vi "PLS Main.vi"() -> ()   [LabVIEW 2014]
doc: "This Continuous Measurement sample project is based on the Queued Message Handler template.\n\nThe Event Handling Loop generates messages based on user interface actions.\n\nThe Message Handling Loop processes messages generated by the Event Handling Loop, or by other messages. There are also Acquisition and Logging message handling loop subVIs, and a chart updating loop."
uses:
  Digital Control/type de test.ctl
  Settings/Settings.ctl
  Acquisition/Hardware Configuration.ctl
  Settings/conversion.ctl
  Logging/Logging Configuration.ctl
  Generation/Hardware Configuration.ctl
  Digital Control/Hardware Configuration.ctl
  controls/PLS UI Data.ctl
  controls/PLS UI State.ctl
  Acquisition/GLB_compteurs.vi
  support/Message Queue/Enqueue Message (Single).vi
  support/GLB_PAmonts.vi
  Digital Control/GLB_Timing.vi
  Acquisition/GLB_Fsave.vi
  support/Message Queue/Enqueue Message (Array).vi
  <vilib>/Utility/error.llb/Error Cluster From Error Code.vi
  <vilib>/ErrorRing/Error Ring.xnode
  Acquisition/PLS Acquisition.lvlib
  Logging/PLS Logging.lvlib
  Settings/PLS Settings.lvlib
  support/User Event - Stop/PLS User Event - Stop.lvlib
  support/Message Queue/PLS Message Queue.lvlib
  Generation/PLS Generation.lvlib
  Digital Control/PLS Digital Control.lvlib
panel:
  in  "Tab":enum32{"Mode manuel", "Lancement cycle"}(tab)
  out "Data":waveform(dbl)[](graph)
  in  "p0.2":bool caption="Eau froide"
  in  "p0.3":bool caption="Eau chaude"
  in  "p0.5":bool caption="Coup de bélier"
  out "compteurs":T1 {"Ligne 4" format="%#.3f l/min"; "Ligne 3" format="%#.3f l/min"; "Ligne 2" format="%#.3f l/min"; "c0" format="%#.3f l/min"}
  in  "Start":bool
  in  "Stop":bool
  in  "Settings":bool
  in  "L4_Twarm":dbl=5.0 caption="Période chaude" min=5.0 max=1000.0 step=0.1 format="%d s"
  in  "L4_Tcold":dbl=5.0 caption="Période froide" min=5.0 max=1000.0 step=0.1 format="%d s"
  in  "L4_Tcons":dbl=30.0 caption="T consigne" min=10.0 max=80.0 step=1.0 format="%#.1f °C"
  in  "L4_stop":bool
  in  "L4_start":bool
  in  "L4_file":path caption="Fichier de sortie"
  in  "L4_fsave":i32(ring)=10 caption="Fréquence enregistrement" items=["1 kHz"=10, "100 Hz"=100, "10 Hz"=1000, "1 Hz"=10000]
  out "Temp":dbl(slide) caption="Température" scale=0.0..100.0
  out "L4_Vtot":dbl caption="Volume total" format="%#.1f l"
  out "L4_debit":dbl(knob) caption="Débit" scale=0.0..15.0
  out "L4_Pfiltre":dbl(knob) caption="Pression filtre" scale=0.0..10.0
  in  "L4_Pamont":dbl=1.0 caption="Pression amont" min=0.0 max=10.0 step=0.1 format="%#.1f Bar"
  in  "Type de test":T2
  out "L3_Vtot":dbl caption="Volume total" format="%#.1f l"
  in  "L3_stop":bool
  in  "L3_start":bool
  in  "L3_file":path caption="Fichier de sortie"
  in  "L3_fsave":i32(ring)=10 caption="Fréquence enregistrement" items=["1 kHz"=10, "100 Hz"=100, "10 Hz"=1000, "1 Hz"=10000]
  out "L3_debit":dbl(knob) caption="Débit" scale=0.0..15.0
  out "L3_Pfiltre":dbl(knob) caption="Pression filtre" scale=0.0..10.0
  in  "L3_Pamont":dbl=1.0 caption="Pression amont" min=0.0 max=10.0 step=0.1 format="%#.1f Bar"
  out "L2_Vtot":dbl caption="Volume total" format="%#.1f l"
  in  "L2_stop":bool
  in  "L2_start":bool
  in  "L2_file":path caption="Fichier de sortie"
  in  "L2_fsave":i32(ring)=10 caption="Fréquence enregistrement" items=["1 kHz"=10, "100 Hz"=100, "10 Hz"=1000, "1 Hz"=10000]
  out "L2_debit":dbl(knob) caption="Débit" scale=0.0..15.0
  out "L2_Pfiltre":dbl(knob) caption="Pression filtre" scale=0.0..10.0
  in  "L2_Pamont":dbl=1.0 caption="Pression amont" min=0.0 max=10.0 step=0.1 format="%#.1f Bar"
  in  "L1_stop":bool
  in  "L1_start":bool
  in  "L1_file":path caption="Fichier de sortie"
  in  "L1_fsave":i32(ring)=10 caption="Fréquence enregistrement" items=["1 kHz"=10, "100 Hz"=100, "10 Hz"=1000, "1 Hz"=10000]
  in  "L1_Tclose":dbl=5.0 caption="Période fermeture" min=5.0 max=1000.0 step=0.1 format="%d s"
  in  "L1_Topen":dbl=5.0 caption="Période ouverture" min=5.0 max=1000.0 step=0.1 format="%d s"
  out "L1_debit":dbl(knob) caption="Débit" scale=0.0..25.0
  out "L1_Pfiltre":dbl(knob) caption="Pression filtre" scale=0.0..15.0
  in  "L1_Pamont":dbl=1.0 caption="Pression amont" min=0.0 max=10.0 step=0.1 format="%#.1f Bar"
  out "soft":string
  # "Ligne 1"
  # "Ligne 2"
  # "Ligne 3"
  # "Ligne 4"
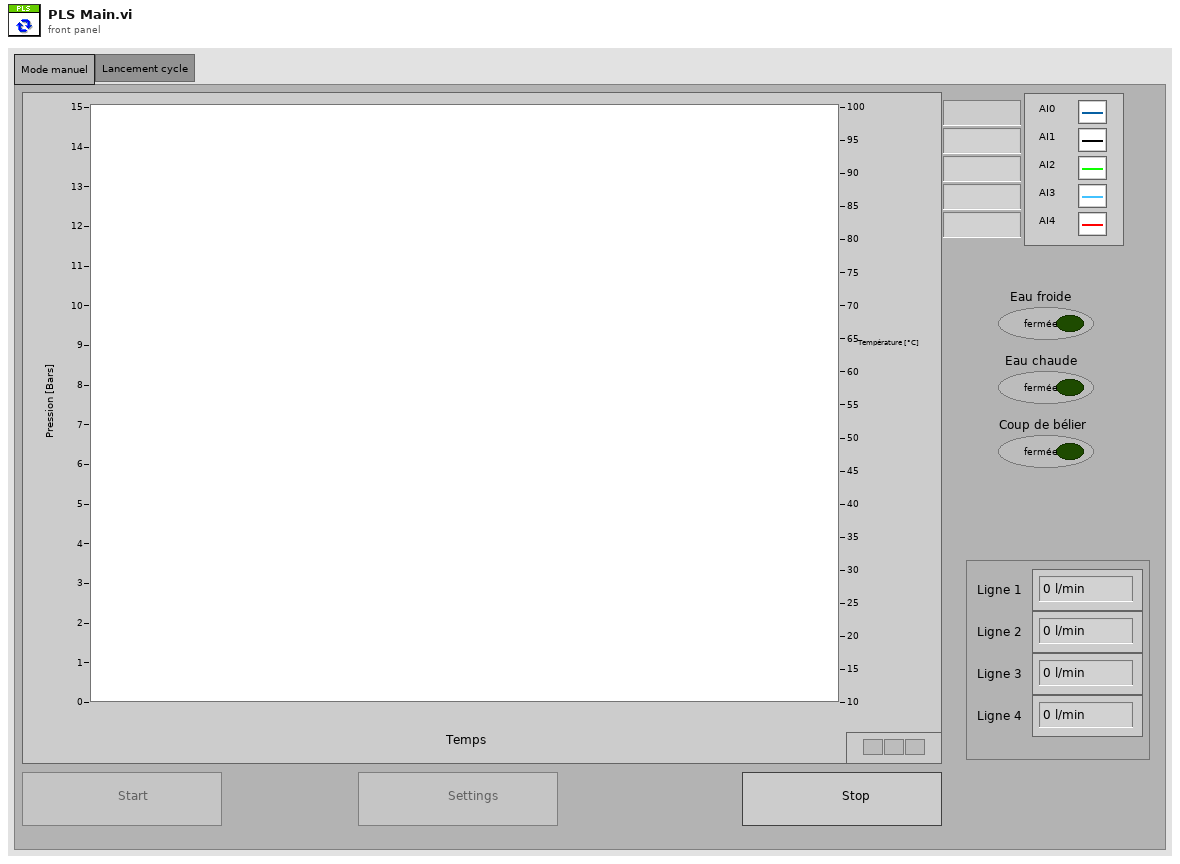
[diagram p1: front panel]
types:
  T1 = cluster{"c0":dbl, "Ligne 2":dbl, "Ligne 3":dbl, "Ligne 4":dbl}
  T2 = typedef "type de test.ctl" = enum16{"Eau froide - standard", "Eau chaude", "Chocs thermiques"}
  T3 = typedef "PLS UI State.ctl" = enum16{"Idle", "Acquiring and Logging", "Waiting for Exit", "Waiting for Exit (Acq Stopped)", "Waiting for Exit (Log Stopped)", "Waiting for Stop", "Waiting for Stop (Acq Stopped)", "Waiting for Stop (Log Stopped)"}
  T4 = typedef "PLS UI Data.ctl" = cluster{"Data Ref":refnum<vi>, "Settings Ref":refnum<vi>, "stop":cluster{"man":refnum<vi>, "L1":refnum<vi>, "L2":refnum<vi>, "L3":refnum<vi>, "L4":refnum<vi>}, "start":cluster{"man":refnum<vi>, "L1":refnum<vi>, "L2":refnum<vi>, "L3":refnum<vi>, "L4":refnum<vi>}, "file":cluster{"L1":refnum<vi>, "L2":refnum<vi>, "L3":refnum<vi>, "L4":refnum<vi>}, "pamont":cluster{"L1":refnum<vi>, "L2":refnum<vi>, "L3":refnum<vi>, "L4":refnum<vi>}, "Fsave":cluster{"L1_fsave":refnum<vi>, "L2_fsave":refnum<vi>, "L3_fsave":refnum<vi>, "L4_fsave":refnum<vi>}, "Tvanne":cluster{"open":refnum<vi>, "close":refnum<vi>}, "Ttemp":cluster{"cold":refnum<vi>, "warm":refnum<vi>}, "temp":refnum<vi>, "Type":refnum<vi>}
  T5 = typedef "PLS Settings.lvlib/Settings.ctl" = cluster{"Acquisition Settings":T6, "Logging Configuration":T8, "Generation Settings":T9, "Digital Control Configuration":T10}
  T6 = typedef "PLS Acquisition.lvlib/Hardware Configuration.ctl" = cluster{"AI":cluster{"task name":string, "task_ref":refnum<k21>, "physical channels":tag, "channels config":cluster{"input terminal configuration":i32, "minimum value":dbl, "maximum value":dbl}, "rate":dbl}, "conversions":cluster{"ai0":T7, "ai1":T7, "ai2":T7, "ai3":T7, "ai4":T7}, "compteur 0":cluster{"task name":string, "task_ref":refnum<k21>, "ctr":tag, "coeff":dbl}, "compteur 1":cluster{"task name":string, "task_ref":refnum<k21>, "ctr":tag, "coeff":dbl}, "compteur 2":cluster{"task name":string, "task_ref":refnum<k21>, "ctr":tag, "coeff":dbl}, "compteur 3":cluster{"task name":string, "task_ref":refnum<k21>, "ctr":tag, "coeff":dbl}}
  T7 = typedef "PLS Settings.lvlib/conversion.ctl" = cluster{"a":dbl, "b":dbl}
  T8 = typedef "PLS Logging.lvlib/Logging Configuration.ctl" = cluster{"Log File Base Path":path, "L1":cluster{"ref":refnum<file>, "actif?":bool, "Fsave":i32}, "L2":cluster{"ref":refnum<file>, "actif?":bool, "Fsave":i32}, "L3":cluster{"ref":refnum<file>, "actif?":bool, "Fsave":i32}, "L4":cluster{"ref":refnum<file>, "actif?":bool, "Fsave":i32}}
  T9 = typedef "PLS Generation.lvlib/Hardware Configuration.ctl" = cluster{"AO":cluster{"task name":string, "task_ref":refnum<k21>, "physical channels":tag}, "PID":cluster{"P":dbl, "I":dbl, "D":dbl}, "conversions":cluster{"ao0":T7}, "setpoint":dbl}
  T10 = typedef "PLS Digital Control.lvlib/Hardware Configuration.ctl" = cluster{"DO":cluster{"task name":string, "task_ref":refnum<k21>, "lines":tag}}
  T11 = typedef "PLS Message Queue.lvlib/All Message Queues.ctl" = cluster{"UI":refnum<queue>, "Acquisition":refnum<queue>, "Logging":refnum<queue>, "Generation":refnum<queue>, "Digital":refnum<queue>}
  T12 = enum8{"Enabled", "Disabled", "Disabled and Grayed Out"}
  T13 = cluster{"L1_Pamont":dbl, "L2_Pamont":dbl, "L3_Pamont":dbl, "L4_Pamont":dbl}
  T14 = cluster{"L1_fsave":i32, "L2_fsave":i32, "L3_fsave":i32, "L4_fsave":i32}
  T15 = enum16{"Eau froide - standard", "Eau chaude", "Chocs thermiques"}
  T16 = cluster{"Stop":refnum<vi>, "L1_stop":refnum<vi>, "L2_stop":refnum<vi>, "L3_stop":refnum<vi>, "L4_stop":refnum<vi>}
  T17 = cluster{"Start":refnum<vi>, "L1_start":refnum<vi>, "L2_start":refnum<vi>, "L3_start":refnum<vi>, "L4_start":refnum<vi>}
  T18 = cluster{"L1_Pamont":refnum<vi>, "L2_Pamont":refnum<vi>, "L3_Pamont":refnum<vi>, "L4_Pamont":refnum<vi>}
  T19 = cluster{"L1_file":refnum<vi>, "L2_file":refnum<vi>, "L3_file":refnum<vi>, "L4_file":refnum<vi>}
  T20 = cluster{"L1_fsave":refnum<vi>, "L2_fsave":refnum<vi>, "L3_fsave":refnum<vi>, "L4_fsave":refnum<vi>}
  T21 = cluster{"L1_Topen":refnum<vi>, "L1_Tclose":refnum<vi>}
  T22 = cluster{"L4_Tcold":refnum<vi>, "L4_Twarm":refnum<vi>}
  T23 = cluster{"man":refnum<vi>, "L1":refnum<vi>, "L2":refnum<vi>, "L3":refnum<vi>, "L4":refnum<vi>}
  T24 = typedef "PLS Logging.lvlib/start info.ctl" = cluster{"path":path, "Fsave":i32, "#ligne":i32}
  T25 = typedef "start info.ctl" = cluster{"type":T2, "ligne index":i32}
  T26 = cluster{"L1":refnum<vi>, "L2":refnum<vi>, "L3":refnum<vi>, "L4":refnum<vi>}
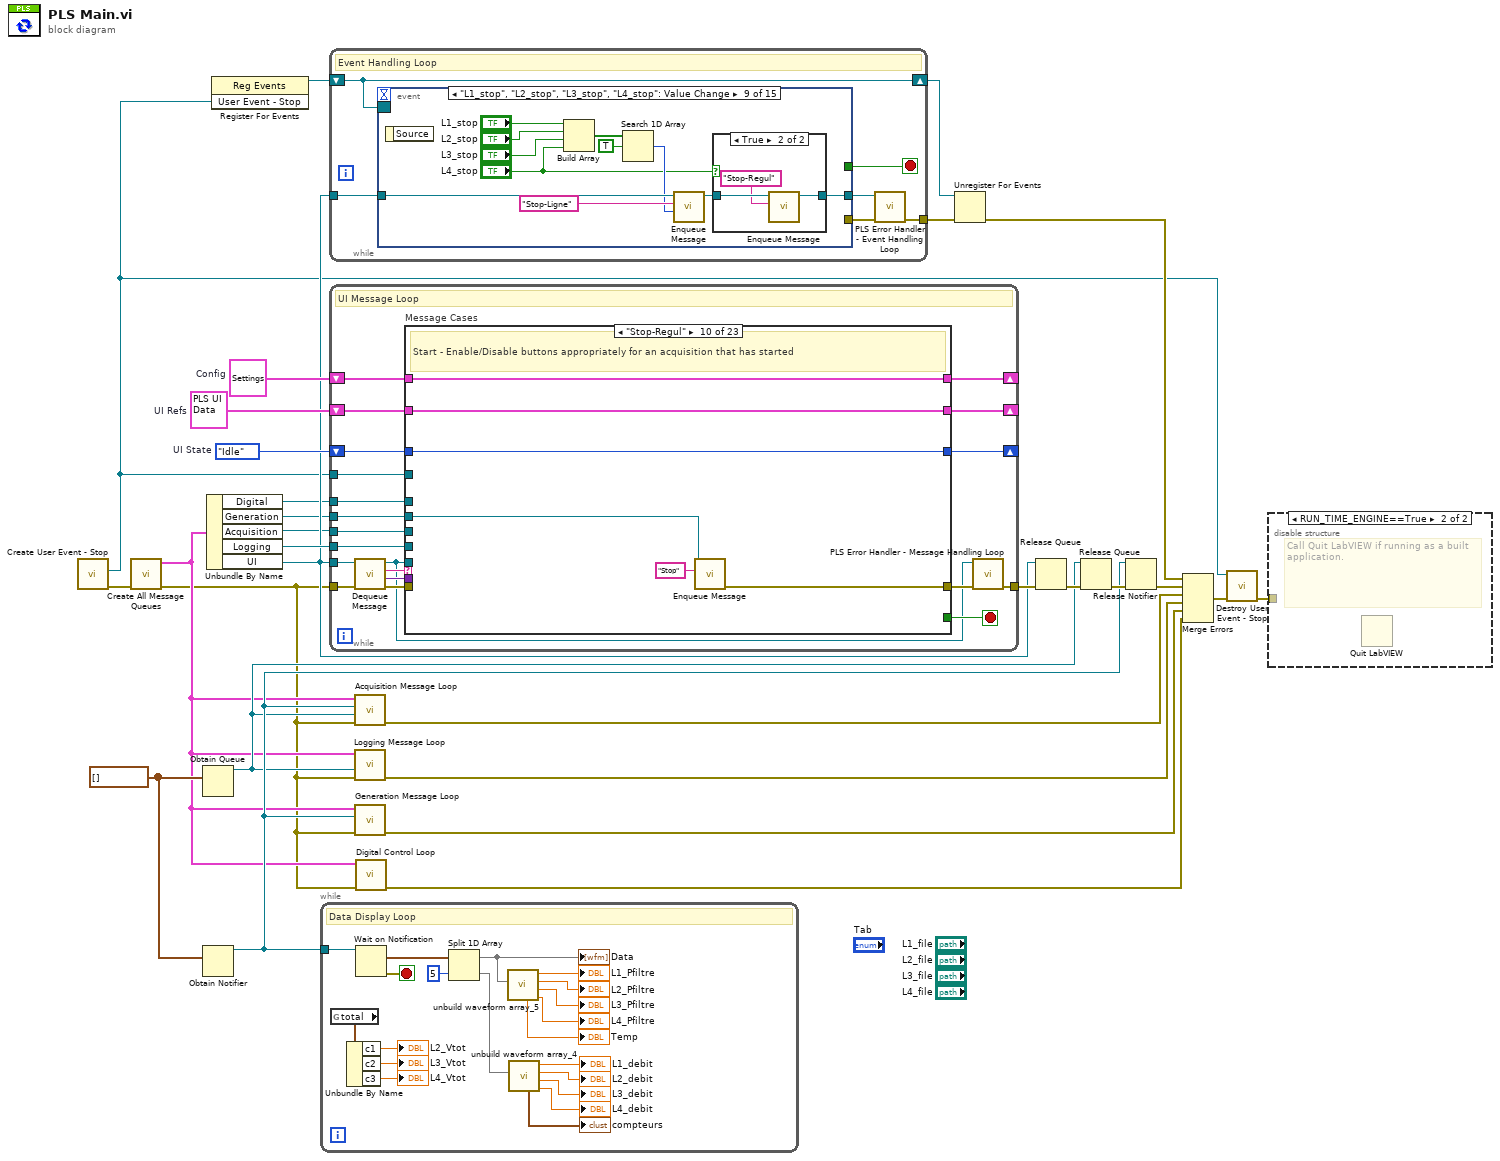
[diagram p0: block diagram]
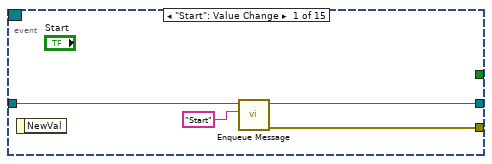
[diagram p3: hidden frame]
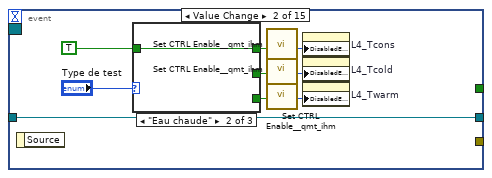
[diagram p4: hidden frame]
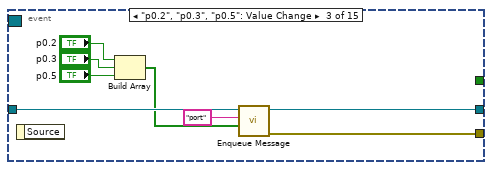
[diagram p7: hidden frame]
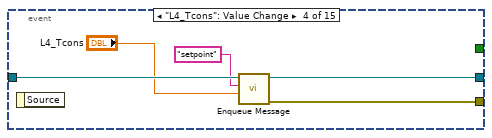
[diagram p8: hidden frame]
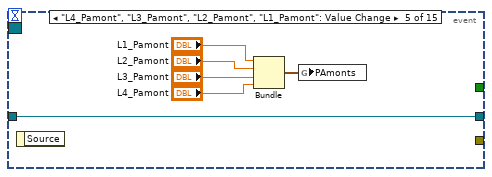
[diagram p9: hidden frame]
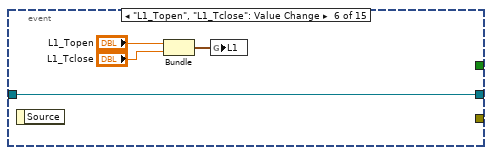
[diagram p10: hidden frame]
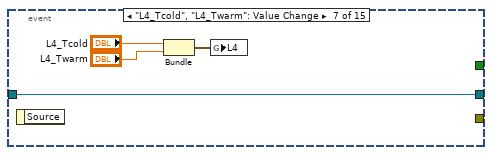
[diagram p11: hidden frame]
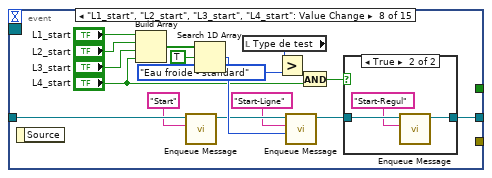
[diagram p12: hidden frame]
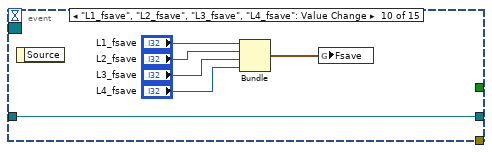
[diagram p15: hidden frame]
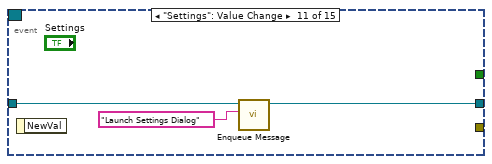
[diagram p16: hidden frame]
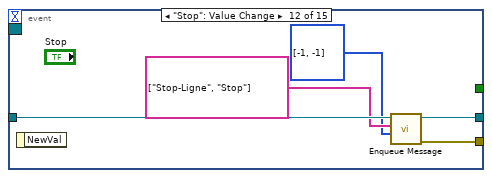
[diagram p17: hidden frame]
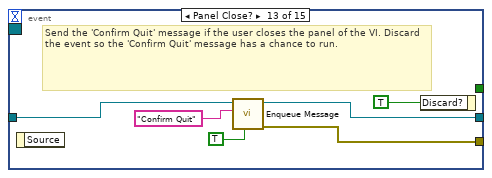
[diagram p18: hidden frame]
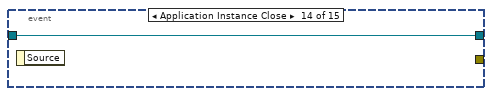
[diagram p19: hidden frame]
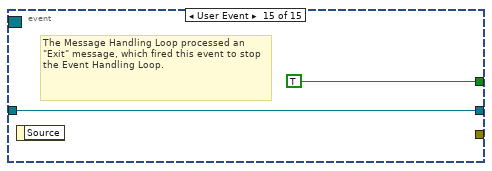
[diagram p20: hidden frame]
diagram:
  w20 = PLS_UI_State."Idle"  # UI State
  w13 = waveform(dbl)[] []
  w22 = T4 {"Data Ref"=refnum, "Settings Ref"=refnum, "stop"={"man"=refnum, "L1"=refnum, "L2"=refnum, "L3"=refnum, "L4"=refnum}, "start"={"man"=refnum, "L1"=refnum, "L2"=refnum, "L3"=refnum, "L4"=refnum}, "file"={"L1"=refnum, "L2"=refnum, "L3"=refnum, "L4"=refnum}, "pamont"={"L1"=refnum, "L2"=refnum, "L3"=refnum, "L4"=refnum}, "Fsave"={"L1_fsave"=refnum, "L2_fsave"=refnum, "L3_fsave"=refnum, "L4_fsave"=refnum}, "Tvanne"={"open"=refnum, "close"=refnum}, "Ttemp"={"cold"=refnum, "warm"=refnum}, "temp"=refnum, "Type"=refnum}  # UI Refs
  w25 = T5 {"Acquisition Settings"={"AI"={"task name"="AI", "task_ref"="", "physical channels"="Dev1/ai0:7", "channels config"={"input terminal configuration"=10106, "minimum value"=-5.0, "maximum value"=5.0}, "rate"=1000.0}, "conversions"={"ai0"={"a"=0.0, "b"=0.0}, "ai1"={"a"=0.0, "b"=0.0}, "ai2"={"a"=0.0, "b"=0.0}, "ai3"={"a"=0.0, "b"=0.0}, "ai4"={"a"=0.0, "b"=0.0}}, "compteur 0"={"task name"="CTR", "task_ref"="", "ctr"="Dev1/ctr0:3", "coeff"=4000.0}, "compteur 1"={"task name"="CTR1", "task_ref"="", "ctr"="Dev1/ctr1", "coeff"=4000.0}, "compteur 2"={"task name"="CTR2", "task_ref"="", "ctr"="Dev1/ctr2", "coeff"=4000.0}, "compteur 3"={"task name"="CTR3", "task_ref"="", "ctr"="Dev1/ctr3", "coeff"=4000.0}}, "Logging Configuration"={"Log File Base Path"=path "", "L1"={"ref"=refnum, "actif?"=FALSE, "Fsave"=0}, "L2"={"ref"=refnum, "actif?"=FALSE, "Fsave"=0}, "L3"={"ref"=refnum, "actif?"=FALSE, "Fsave"=0}, "L4"={"ref"=refnum, "actif?"=FALSE, "Fsave"=0}}, "Generation Settings"={"AO"={"task name"="AO", "task_ref"="", "physical channels"="Dev1/ao0"}, "PID"={"P"=0.0, "I"=0.0, "D"=0.0}, "conversions"={"ao0"={"a"=0.0, "b"=0.0}}, "setpoint"=0.0}, "Digital Control Configuration"={"DO"={"task name"="DO", "task_ref"="", "lines"="Dev1/port0/line2:3, Dev1/port0/line5"}}}  # Config
  n1 = call "Create User Event - Stop.vi"() -> ("error out"=w26:errorcluster, "User Event - Stop"=w1:refnum<user-event>)  [unwired: 10 in]
  n2 = call "Create All Message Queues.vi"("error in (no error)"=w26) -> ("error out"=w3:errorcluster, "Message Queues out"=w4:T11)  [unwired: 9 in]
  n3 = Obtain Queue(element data type=w13) -> (queue out=w11:refnum<queue>)  [unwired: 4 in, 2 out]
  n4 = Obtain Notifier(notification data type=w13) -> (notifier out=w12:refnum<notifier>)  [unwired: 3 in, 2 out]
  n5 = Unbundle By Name(w4) -> ("Digital"=w5:refnum<queue>, "Generation"=w6:refnum<queue>, "Acquisition"=w7:refnum<queue>, "Logging"=w21:refnum<queue>, "UI"=w18:refnum<queue>)
  n6 = register-events(w1) -> (reference out=w10:refnum<event-registration>)  [unwired: 2 in, 1 out]
  n7 = while "Data Display Loop" {
    tunnel: w12 -> [w49]
    stop <- w48 stop-if-true
    # "Data Display Loop"
    n8 = global read "GLB_compteurs.vi" "total"() -> (w33:cluster{"c0":dbl, "c1":dbl, "c2":dbl, "c3":dbl})
    n9 = Unbundle By Name(w33) -> ("c1"=→"L2_Vtot":dbl, "c2"=→"L3_Vtot":dbl, "c3"=→"L4_Vtot":dbl)
    n10 = Wait on Notification(notifier=w49) -> (notification=w46:waveform(dbl)[], error out=w48:errorcluster)  [unwired: 3 in, 2 out]
    n11 = Split 1D Array(array=w46, index=5) -> (first subarray=w42:waveform(dbl)[], second subarray=w39:waveform(dbl)[])
    "Data" <- w42
    n12 = call "unbuild waveform array_5.vi"("Array"=w42) -> ("l4"=→"L4_Pfiltre":dbl, "l3"=→"L3_Pfiltre":dbl, "l2"=→"L2_Pfiltre":dbl, "l1"=→"L1_Pfiltre":dbl, "t"=→"Temp":dbl)  [unwired: 6 in]
    n13 = call "unbuild waveform array_4.vi"("Array"=w39) -> ("4"=→"L4_debit":dbl, "3"=→"L3_debit":dbl, "2"=→"L2_debit":dbl, "1"=→"L1_debit":dbl, "débits"=→"compteurs":cluster{dbl, dbl, dbl, dbl})  [unwired: 6 in]
  }
  n14 = while {
    tunnel: w18 -> [w55]
    tunnel: [w53] -> w28
    shift-right: [w50] -> w23
    shift-left: w10 -> [w50]
    stop <- w54 stop-if-true
    # "Event Handling Loop"
    n15 = event shown="[8] \"L1_stop\", \"L2_stop\", \"L3_stop\", \"L4_stop\": Value Change" {
      selector: w50 -> [_ _ _ _ _ _ _ _ _ _ _ _ _ _ _]
      dyn-events: _ -> [_ _ _ _ _ _ _ _ _ _ _ _ _ _ _]
      timeout: _ -> [_ _ _ _ _ _ _ _ _ _ _ _ _ _ _]
      tunnel: [_ _ _ _ _ _ _ _ _ _ _ _ _ _ TRUE ("Discard?")] -> w54
      tunnel: w55 -> [w59 w68 w78 w83 w89 w93 w97 w107 w128 w134 w141 w147 w151 w154 w155]
      tunnel: [w57 _ w77 w82 _ _ _ _ _ _ _ w146 w149 _ _] -> w52
      tunnel: [w56 w68 w76 w81 w89 w93 w97 w104 w120 w134 w140 w145 w150 w154 w155] -> w51
      event "Start": Value Change {
        n16 = event-data() -> ()  [unwired: 1 in, 1 out]
        n17 = call-poly "Enqueue Message.vi"("Message"="Start", "Message Queue"=w59) -> ("error out"=w57:errorcluster, "dup Message Queue"=w56:refnum<queue>)  [unwired: 8 in]
      }
      event Value Change {
        n18 = event-data() -> ()  [unwired: 1 in, 1 out]
        n19 = case shown="\"Eau chaude\"" "Type de test" {
          tunnel: [_ w69 w70] -> w65
          tunnel: [_ _ w70] -> w64
          tunnel: [_ _ w70] -> w63
          tunnel: TRUE ("set disable?") -> [_ w69 w70]
          frame "Eau froide - standard" {
          }
          frame "Eau chaude" {
          }
          frame "Chocs thermiques" {
          }
        }
        n20 = call <userlib>:"Set CTRL Enable__qmt_ihm.vi"("set enable?"=w65) -> ("Disable?"=w66:T12)  [unwired: 6 in]
        n21 = call <userlib>:"Set CTRL Enable__qmt_ihm.vi"("set enable?"=w64) -> ("Disable?"=w62:T12)  [unwired: 6 in]
        n22 = call <userlib>:"Set CTRL Enable__qmt_ihm.vi"("set enable?"=w63) -> ("Disable?"=w61:T12)  [unwired: 6 in]
        n23 = property on="L4_Tcons" class="DigNum (strict)"("DisabledEnum"=w66) -> ()  [unwired: 2 in, 2 out]
        n24 = property on="L4_Tcold" class="DigNum (strict)"("DisabledEnum"=w62) -> ()  [unwired: 2 in, 2 out]
        n25 = property on="L4_Twarm" class="DigNum (strict)"("DisabledEnum"=w61) -> ()  [unwired: 2 in, 2 out]
      }
      event "p0.2", "p0.3", "p0.5": Value Change {
        n26 = event-data() -> ()  [unwired: 1 in, 1 out]
        n27 = Build Array("p0.2", "p0.3", "p0.5") -> (w73:bool[])
        n28 = call-poly "Enqueue Message.vi"("Message Data"=w73, "Message"="port", "Message Queue"=w78) -> ("error out"=w77:errorcluster, "dup Message Queue"=w76:refnum<queue>)  [unwired: 7 in]
      }
      event "L4_Tcons": Value Change {
        n29 = event-data() -> ()  [unwired: 1 in, 1 out]
        n30 = call-poly "Enqueue Message.vi"("Message Data"="L4_Tcons", "Message"="setpoint", "Message Queue"=w83) -> ("error out"=w82:errorcluster, "dup Message Queue"=w81:refnum<queue>)  [unwired: 7 in]
      }
      event "L4_Pamont", "L3_Pamont", "L2_Pamont", "L1_Pamont": Value Change {
        n31 = event-data() -> ()  [unwired: 1 in, 1 out]
        n32 = Bundle("L1_Pamont"="L1_Pamont", "L2_Pamont"="L2_Pamont", "L3_Pamont"="L3_Pamont", "L4_Pamont"="L4_Pamont") -> (w84:T13)  [unwired: 1 in]
        n33 = global write "GLB_PAmonts.vi" "PAmonts"(w84) -> ()
      }
      event "L1_Topen", "L1_Tclose": Value Change {
        n34 = event-data() -> ()  [unwired: 1 in, 1 out]
        n35 = Bundle("L1_Topen"="L1_Topen", "L1_Tclose"="L1_Tclose") -> (w90:cluster{"L1_Topen":dbl, "L1_Tclose":dbl})  [unwired: 1 in]
        n36 = global write "GLB_Timing.vi" "L1"(w90) -> ()
      }
      event "L4_Tcold", "L4_Twarm": Value Change {
        n37 = event-data() -> ()  [unwired: 1 in, 1 out]
        n38 = Bundle("L4_Tcold"="L4_Tcold", "L4_Twarm"="L4_Twarm") -> (w96:cluster{"L4_Tcold":dbl, "L4_Twarm":dbl})  [unwired: 1 in]
        n39 = global write "GLB_Timing.vi" "L4"(w96) -> ()
      }
      event "L1_start", "L2_start", "L3_start", "L4_start": Value Change {
        n40 = event-data() -> ()  [unwired: 1 in, 1 out]
        n41 = Build Array("L1_start", "L2_start", "L3_start", "L4_start") -> (w111:bool[])
        n42 = call-poly "Enqueue Message.vi"("Message"="Start", "Message Queue"=w107) -> ("dup Message Queue"=w108:refnum<queue>)  [unwired: 8 in, 1 out]
        n43 = Search 1D Array(1D array=w111, element=TRUE) -> (index of element=w109:i32)  [unwired: 1 in]
        n44 = local read "Type de test"() -> (w101:T2)
        n45 = Greater?(x=w101, y=type_de_test."Eau froide - standard") -> (0:w99:bool)
        n46 = call-poly "Enqueue Message.vi"("Message Data"=w109, "Message"="Start-Ligne", "Message Queue"=w108) -> ("dup Message Queue"=w105:refnum<queue>)  [unwired: 7 in, 1 out]
        n47 = And(x=w99, y="L4_start") -> (x .and. y?=w103:bool)
        n48 = case shown="True" w103 {
          tunnel: w105 -> [w115 w118]
          tunnel: [w115 w117] -> w104
          frame False {
          }
          frame True {
            n49 = call-poly "Enqueue Message.vi"("Message"="Start-Regul", "Message Queue"=w118) -> ("dup Message Queue"=w117:refnum<queue>)  [unwired: 8 in, 1 out]
          }
        }
      }
      event "L1_stop", "L2_stop", "L3_stop", "L4_stop": Value Change {
        n50 = event-data() -> ()  [unwired: 1 in, 1 out]
        n51 = Build Array("L1_stop", "L2_stop", "L3_stop", "L4_stop") -> (w127:bool[])
        n52 = Search 1D Array(1D array=w127, element=TRUE) -> (index of element=w125:i32)  [unwired: 1 in]
        n53 = call-poly "Enqueue Message.vi"("Message Data"=w125, "Message"="Stop-Ligne", "Message Queue"=w128) -> ("dup Message Queue"=w121:refnum<queue>)  [unwired: 7 in, 1 out]
        n54 = case shown="True" "L4_stop" {
          tunnel: w121 -> [w130 w133]
          tunnel: [w130 w132] -> w120
          frame False {
          }
          frame True {
            n55 = call-poly "Enqueue Message.vi"("Message"="Stop-Regul", "Message Queue"=w133) -> ("dup Message Queue"=w132:refnum<queue>)  [unwired: 8 in, 1 out]
          }
        }
      }
      event "L1_fsave", "L2_fsave", "L3_fsave", "L4_fsave": Value Change {
        n56 = event-data() -> ()  [unwired: 1 in, 1 out]
        n57 = Bundle("L1_fsave"="L1_fsave", "L2_fsave"="L2_fsave", "L3_fsave"="L3_fsave", "L4_fsave"="L4_fsave") -> (w138:T14)  [unwired: 1 in]
        n58 = global write "GLB_Fsave.vi" "Fsave"(w138) -> ()
      }
      event "Settings": Value Change {
        n59 = event-data() -> ()  [unwired: 1 in, 1 out]
        n60 = call-poly "Enqueue Message.vi"("Message"="Launch Settings Dialog", "Message Queue"=w141) -> ("dup Message Queue"=w140:refnum<queue>)  [unwired: 8 in, 1 out]
      }
      event "Stop": Value Change {
        n61 = event-data() -> ()  [unwired: 1 in, 1 out]
        n62 = call-poly "Enqueue Message.vi"("Message Data Array"=i32[] [-1, -1], "Message Array"=string[] ["Stop-Ligne", "Stop"], "Message Queue"=w147) -> ("error out"=w146:errorcluster, "dup Message Queue"=w145:refnum<queue>)  [unwired: 7 in]
      }
      event Panel Close? {
        # "Send the 'Confirm Quit' message if the user closes the panel of the VI. Discard the event so the 'Confirm Quit' message has a chance to run."
        n63 = event-data() -> ()  [unwired: 1 in, 1 out]
        n64 = call-poly "Enqueue Message.vi"("Priority Message? (F)"=TRUE, "Message"="Confirm Quit", "Message Queue"=w151) -> ("error out"=w149:errorcluster, "dup Message Queue"=w150:refnum<queue>)  [unwired: 7 in]
        n65 = event-data("Discard?"=TRUE) -> ()  [unwired: 1 in, 1 out]
      }
      event Application Instance Close {
        n66 = event-data() -> ()  [unwired: 1 in, 1 out]
      }
      event User Event {
        # "The Message Handling Loop processed an \"Exit\" message, which fired this event to stop the Event Handling Loop."
        n67 = event-data() -> ()  [unwired: 1 in, 1 out]
      }
    }
    n68 = call "PLS Error Handler - Event Handling Loop.vi"("error in (no error)"=w52, "Message Queue"=w51) -> ("dup error in"=w53:errorcluster)  [unwired: 8 in, 1 out]
  }
  n69 = while {
    tunnel: w18 -> [w170]
    tunnel: w1 -> [w175]
    shift-right: [w169] -> _
    shift-left: w25 -> [w168]
    shift-right: [w166] -> _
    shift-left: w22 -> [w167]
    tunnel: w7 -> [w165]
    tunnel: w21 -> [w164]
    shift-right: [w159] -> _
    shift-left: w20 -> [w160]
    tunnel: w3 -> [w174]
    tunnel: [w163] -> w29
    tunnel: w6 -> [w158]
    tunnel: w5 -> [w157]
    stop <- w176 stop-if-true
    # "UI Message Loop"
    n70 = call "Dequeue Message.vi"("error in (no error)"=w174, "Message Queue"=w170) -> ("error out"=w173:errorcluster, "Message Data"=w171:variant, "Message"=w172:string, "dup Message Queue"=w161:refnum<queue>)  [unwired: 6 in]
    n71 = case "Message Cases" shown="\"Stop-Regul\"" w172 {
      selector: w172 -> [_ _ _ _ _ _ w267 w287 _ _ w316 w328 _ _ _ _ _ _ w456 _ w480 w488 w494]
      tunnel: w161 -> [w186 _ _ _ _ _ _ _ _ _ _ _ w351 w372 _ w416 w431 w440 _ _ _ _ _]
      tunnel: w173 -> [w185 w209 w229 w247 w260 w266 w270 _ _ _ _ _ w352 w373 _ w418 _ w439 _ w476 w478 w486 _]
      tunnel: [w178 w209 w229 w247 w260 w266 w272 w290 w303 w309 w318 w346 w349 w370 w392 w411 w430 w438 w469 w475 w482 w490 w493] -> w162
      tunnel: [_ _ _ _ _ _ _ _ _ _ _ _ _ _ _ _ _ _ TRUE _ _ _ _] -> w176
      tunnel: w171 -> [_ _ _ _ _ _ _ w298 _ _ w325 _ _ _ _ _ w432 _ _ _ w479 w487 _]
      tunnel: w175 -> [_ _ _ _ _ _ _ _ _ _ _ _ _ _ _ _ _ _ w470 _ _ _ _]
      tunnel: [w188 w208 w228 w246 w259 w262 w283 w300 w306 w312 w327 w345 w355 w376 w408 w415 w436 w443 w468 w474 w484 w492 w497] -> w169
      tunnel: w168 -> [w189 w208 w228 w246 w259 w262 w283 w300 w306 w312 w327 w345 w355 w376 w408 w419 w436 w443 w468 w474 w484 w492 w497]
      tunnel: w167 -> [w187 w207 w224 w244 w257 w265 w282 w299 w305 w311 w326 w344 w354 w375 w402 w413 w435 w442 w467 w473 w483 w491 w496]
      tunnel: [w187 w202 w226 w231 w257 w265 w282 w299 w305 w311 w326 w344 w354 w375 w402 w413 w435 w442 w467 w473 w483 w491 w496] -> w166
      tunnel: w165 -> [_ _ _ _ _ _ w274 w288 _ _ w317 w336 _ _ w405 _ _ _ w458 _ _ _ _]
      tunnel: w164 -> [_ _ _ _ _ _ _ w292 _ _ w320 _ _ _ _ _ _ _ w460 _ _ _ _]
      tunnel: w160 -> [_ _ _ _ _ w264 _ w296 w304 w310 w323 w334 w353 w374 w406 w412 w428 w441 _ w472 w481 w489 w495]
      tunnel: [PLS_UI_State."Idle" ("UI State") PLS_UI_State."Idle" ("UI State") PLS_UI_State."Idle" ("UI State") PLS_UI_State."Idle" ("UI State") PLS_UI_State."Idle" ("UI State") w264 PLS_UI_State."Acquiring and Logging" ("UI State") w296 w304 w310 w323 w335 w350 w371 w406 w412 w428 w437 PLS_UI_State."Idle" ("UI State") w472 w481 w489 w495] -> w159
      tunnel: w158 -> [_ _ _ _ _ _ _ _ w301 w307 _ w333 _ _ w404 _ _ _ w459 _ _ w485 _]
      tunnel: w157 -> [_ _ _ _ _ _ w271 w293 _ _ w321 w332 _ _ w397 _ _ _ w457 _ w477 _ _]
      frame "Initialize" {
        # "Initialize - Get configuration settings, then message the UI to initialize, and broadcast the settings to the other message loops."
        n72 = call-poly "Enqueue Message.vi"("error in (no error)"=w185, "Message Array"=string[] ["Init Refs 1", "Init Refs 2", "Init Refs 3", "Init UI", "Default values", "Broadcast Settings"], "Message Queue"=w186) -> ("error out"=w177:errorcluster)  [unwired: 7 in, 1 out]
        n73 = control-ref of="?"() -> (w181:refnum<vi>)
        n74 = call "Load Settings from XML.vi"("Settings in"=w189) -> ("Settings out"=w188:T5)  [unwired: 9 in, 1 out]
        n75 = call "AppKind.vi"("VI in"=w181) -> ("File Version Info"=w182:string)  [unwired: 10 in]
        n76 = Concatenate Strings("PLS Moniteur " ("string"), w182) -> (→"soft":string)
        n77 = Merge Errors(w177) -> (w178:errorcluster)
      }
      frame "Init Refs 1" {
        # "Init UI Refs - Store control references for UI controls.  Also enable/disable controls appropriately."
        n78 = control-ref of="Data"() -> (w206:refnum<vi>)
        n79 = control-ref of="Settings"() -> (w205:refnum<vi>)
        n80 = control-ref of="Stop"() -> (w201:refnum<vi>)
        n81 = control-ref of="L1_stop"() -> (w200:refnum<vi>)
        n82 = control-ref of="L2_stop"() -> (w199:refnum<vi>)
        n83 = control-ref of="L3_stop"() -> (w198:refnum<vi>)
        n84 = control-ref of="L4_stop"() -> (w197:refnum<vi>)
        n85 = Bundle By Name(cluster=w207, "Settings Ref"=w205, "Data Ref"=w206) -> (w203:T4)
        n86 = Bundle("Stop"=w201, "L1_stop"=w200, "L2_stop"=w199, "L3_stop"=w198, "L4_stop"=w197) -> (w196:T16)  [unwired: 1 in]
        n87 = control-ref of="Start"() -> (w195:refnum<vi>)
        n88 = control-ref of="L1_start"() -> (w194:refnum<vi>)
        n89 = control-ref of="L2_start"() -> (w193:refnum<vi>)
        n90 = control-ref of="L3_start"() -> (w192:refnum<vi>)
        n91 = control-ref of="L4_start"() -> (w191:refnum<vi>)
        n92 = Bundle("Start"=w195, "L1_start"=w194, "L2_start"=w193, "L3_start"=w192, "L4_start"=w191) -> (w190:T17)  [unwired: 1 in]
        n93 = Bundle By Name(cluster=w203, "stop"=w196, "start"=w190) -> (w202:T4)
      }
      frame "Init Refs 2" {
        # "Init UI Refs - Store control references for UI controls.  Also enable/disable controls appropriately."
        n94 = control-ref of="L1_file"() -> (w223:refnum<vi>)
        n95 = control-ref of="L2_file"() -> (w222:refnum<vi>)
        n96 = control-ref of="L3_file"() -> (w221:refnum<vi>)
        n97 = control-ref of="L4_file"() -> (w220:refnum<vi>)
        n98 = control-ref of="L1_Pamont"() -> (w219:refnum<vi>)
        n99 = control-ref of="L2_Pamont"() -> (w218:refnum<vi>)
        n100 = control-ref of="L3_Pamont"() -> (w217:refnum<vi>)
        n101 = control-ref of="L4_Pamont"() -> (w216:refnum<vi>)
        n102 = Bundle("L1_Pamont"=w219, "L2_Pamont"=w218, "L3_Pamont"=w217, "L4_Pamont"=w216) -> (w215:T18)  [unwired: 1 in]
        n103 = Bundle("L1_file"=w223, "L2_file"=w222, "L3_file"=w221, "L4_file"=w220) -> (w225:T19)  [unwired: 1 in]
        n104 = control-ref of="L1_fsave"() -> (w213:refnum<vi>)
        n105 = control-ref of="L2_fsave"() -> (w212:refnum<vi>)
        n106 = control-ref of="L3_fsave"() -> (w211:refnum<vi>)
        n107 = control-ref of="L4_fsave"() -> (w210:refnum<vi>)
        n108 = Bundle("L1_fsave"=w213, "L2_fsave"=w212, "L3_fsave"=w211, "L4_fsave"=w210) -> (w214:T20)  [unwired: 1 in]
        n109 = Bundle By Name(cluster=w224, "file"=w225, "pamont"=w215, "Fsave"=w214) -> (w226:T4)
      }
      frame "Init Refs 3" {
        w230 = FALSE ("start?")
        # "Init UI Refs - Store control references for UI controls.  Also enable/disable controls appropriately."
        n110 = control-ref of="L1_Topen"() -> (w243:refnum<vi>)
        n111 = control-ref of="L1_Tclose"() -> (w242:refnum<vi>)
        n112 = control-ref of="L4_Tcold"() -> (w240:refnum<vi>)
        n113 = control-ref of="L4_Twarm"() -> (w239:refnum<vi>)
        n114 = control-ref of="L4_Tcons"() -> (w237:refnum<vi>)
        n115 = control-ref of="Type de test"() -> (w236:refnum<vi>)
        n116 = Bundle("L1_Topen"=w243, "L1_Tclose"=w242) -> (w241:T21)  [unwired: 1 in]
        n117 = Bundle("L4_Tcold"=w240, "L4_Twarm"=w239) -> (w238:T22)  [unwired: 1 in]
        n118 = Bundle By Name(cluster=w244, "Tvanne"=w241, "Ttemp"=w238, "temp"=w237, "Type"=w236) -> (w231:T4)
        n119 = call "set UI state when start line.vi"("start?"=w230, "index of element"=0, "UI Refs"=w231) -> ()  [unwired: 7 in, 2 out]
        n120 = call "set UI state when start line.vi"("start?"=w230, "index of element"=1, "UI Refs"=w231) -> ()  [unwired: 7 in, 2 out]
        n121 = call "set UI state when start line.vi"("start?"=w230, "index of element"=2, "UI Refs"=w231) -> ()  [unwired: 7 in, 2 out]
        n122 = call "set UI state when start line.vi"("start?"=w230, "index of element"=3, "UI Refs"=w231) -> ()  [unwired: 7 in, 2 out]
      }
      frame "Init UI" {
        # "Init UI Refs - Store control references for UI controls.  Also enable/disable controls appropriately."
        n123 = Unbundle By Name(w257) -> ("Settings Ref"=w252:refnum<vi>, "Data Ref"=w251:refnum<vi>, "start"=w255:T23, "stop"=w250:T23)
        n124 = Cluster To Array(cluster=w255) -> (array=w249:refnum<vi>[])
        n125 = Cluster To Array(cluster=w250) -> (array=w248:refnum<vi>[])
        n126 = Build Array (concatenate)(w252, w251, w249) -> (w254:refnum<vi>[])
        n127 = call "PLS Set Enable State on Multiple Controls.vi"("Enable?"=TRUE, "Controls"=w254) -> ()  [unwired: 10 in]
        n128 = call "PLS Set Enable State on Multiple Controls.vi"("Enable?"=FALSE, "Controls"=w248) -> ()  [unwired: 10 in]
      }
      frame "Default values" {
        # "Init UI Refs - Store control references for UI controls.  Also enable/disable controls appropriately."
        n129 = invoke on="Tab" class="TabCtl (strict)" method="Reinit To Default"() -> ()  [unwired: 3 in, 3 out]
        n130 = property on="Type de test" class="Enum (strict)"("Val(Sgnl)"=T15."Eau froide - standard" ("Value (Signaling)")) -> ()  [unwired: 2 in, 2 out]
        n131 = invoke on="p0.5" class="Bool (strict)" method="Reinit To Default"() -> ()  [unwired: 3 in, 3 out]
        n132 = invoke on="p0.2" class="Bool (strict)" method="Reinit To Default"() -> ()  [unwired: 3 in, 3 out]
        n133 = invoke on="p0.3" class="Bool (strict)" method="Reinit To Default"() -> ()  [unwired: 3 in, 3 out]
        n134 = property on="Data" class="WFChart (strict)"("History Data"=waveform(dbl)[][] []) -> ()  [unwired: 2 in, 2 out]
      }
      frame "Start" {
        # "Start - Enable/Disable buttons appropriately for an acquisition that has started"
        n135 = Unbundle By Name(w282) -> ("stop.man"=w277:refnum<vi>, "start.man"=w276:refnum<vi>, "Settings Ref"=w275:refnum<vi>)
        n136 = Build Array(w276, w275) -> (w280:refnum<vi>[])
        n137 = Build Array(w277) -> (w279:refnum<vi>[])
        n138 = call-poly "Enqueue Message.vi"("Message"=w267, "Message Queue"=w274) -> ("error out"=w269:errorcluster)  [unwired: 8 in, 1 out]
        n139 = call "PLS Set Enable State on Multiple Controls.vi"("Enable?"=TRUE, "Controls"=w279) -> ()  [unwired: 10 in]
        n140 = call "PLS Set Enable State on Multiple Controls.vi"("Enable?"=FALSE, "Controls"=w280) -> ()  [unwired: 10 in]
        n141 = call-poly "Enqueue Message.vi"("Message"=w267, "Message Queue"=w271) -> ("error out"=w268:errorcluster)  [unwired: 8 in, 1 out]
        n142 = Merge Errors(w268, w269, w270) -> (w272:errorcluster)
      }
      frame "Start-Ligne" {
        # "Start - Enable/Disable buttons appropriately for an acquisition that has started"
        n143 = Variant To Data(type=-1 ("index of element"), Variant=w298) -> (data=w284:i32)  [unwired: 1 in, 1 out]
        n144 = call "set UI state when start line.vi"("start?"=TRUE, "index of element"=w284, "UI Refs"=w299) -> ("start info - logging loop"=w294:T24, "start info - digital control loop"=w289:T25)  [unwired: 7 in]
        n145 = call-poly "Enqueue Message.vi"("Message Data"=w294, "Message"=w287, "Message Queue"=w292) -> ("error out"=w286:errorcluster)  [unwired: 7 in, 1 out]
        n146 = call-poly "Enqueue Message.vi"("Message Data"=w284, "Message"=w287, "Message Queue"=w288) -> ("error out"=w285:errorcluster)  [unwired: 7 in, 1 out]
        n147 = call-poly "Enqueue Message.vi"("Message Data"=w289, "Message"=w287, "Message Queue"=w293) -> ("error out"=w291:errorcluster)  [unwired: 7 in, 1 out]
        n148 = Merge Errors(w291, w285, w286) -> (w290:errorcluster)
      }
      frame "Start-Regul" {
        # "Start - Enable/Disable buttons appropriately for an acquisition that has started"
        n149 = call-poly "Enqueue Message.vi"("Message"="Start", "Message Queue"=w301) -> ("error out"=w303:errorcluster)  [unwired: 8 in, 1 out]
      }
      frame "Stop-Regul" {
        # "Start - Enable/Disable buttons appropriately for an acquisition that has started"
        n150 = call-poly "Enqueue Message.vi"("Message"="Stop", "Message Queue"=w307) -> ("error out"=w309:errorcluster)  [unwired: 8 in, 1 out]
      }
      frame "Stop-Ligne" {
        # "Stop - Enable/Disable buttons appropriately for an acquisition that has started"
        n151 = Variant To Data(type=-1 ("index of element"), Variant=w325) -> (data=w315:i32)  [unwired: 1 in, 1 out]
        n152 = call "set UI state when start line.vi"("start?"=FALSE, "index of element"=w315, "UI Refs"=w326) -> ()  [unwired: 7 in, 2 out]
        n153 = call-poly "Enqueue Message.vi"("Message Data"=w315, "Message"=w316, "Message Queue"=w320) -> ("error out"=w314:errorcluster)  [unwired: 7 in, 1 out]
        n154 = call-poly "Enqueue Message.vi"("Message Data"=w315, "Message"=w316, "Message Queue"=w317) -> ("error out"=w313:errorcluster)  [unwired: 7 in, 1 out]
        n155 = call-poly "Enqueue Message.vi"("Message Data"=w315, "Message"=w316, "Message Queue"=w321) -> ("error out"=w319:errorcluster)  [unwired: 7 in, 1 out]
        n156 = Merge Errors(w319, w313, w314) -> (w318:errorcluster)
      }
      frame "Stop" {
        # "Stop - Enable/Disable buttons appropriately for an acquisition that has stopped"
        n157 = Unbundle By Name(w344) -> ("stop.man"=w339:refnum<vi>, "start.man"=w338:refnum<vi>, "Settings Ref"=w337:refnum<vi>)
        n158 = call-poly "Enqueue Message.vi"("Message"=w328, "Message Queue"=w336) -> ("error out"=w331:errorcluster)  [unwired: 8 in, 1 out]
        n159 = Build Array(w338, w337) -> (w342:refnum<vi>[])
        n160 = Build Array(w339) -> (w341:refnum<vi>[])
        n161 = call-poly "Enqueue Message.vi"("Message"=w328, "Message Queue"=w333) -> ("error out"=w330:errorcluster)  [unwired: 8 in, 1 out]
        n162 = call "PLS Set Enable State on Multiple Controls.vi"("Enable?"=FALSE, "Controls"=w341) -> ()  [unwired: 10 in]
        n163 = call "PLS Set Enable State on Multiple Controls.vi"("Enable?"=TRUE, "Controls"=w342) -> ()  [unwired: 10 in]
        n164 = call-poly "Enqueue Message.vi"("Message"=w328, "Message Queue"=w332) -> ("error out"=w329:errorcluster)  [unwired: 8 in, 1 out]
        n165 = case shown="\"Waiting for Exit\"" w334 {
          selector: w334 -> [w347 _]
          tunnel: [w347 PLS_UI_State."Waiting for Stop" ("UI State")] -> w335
          frame "Waiting for Exit" {
          }
          frame Default {
          }
        }
        n166 = Merge Errors(w329, w330, w331) -> (w346:errorcluster)
      }
      frame "Acquisition Stopped" {
        # "Logic for determining what action to take when the acquisition has stopped."
        n167 = case shown="\"Waiting for Exit (Log Stopped)\"" w353 {
          selector: w353 -> [w357 _ _ _ _]
          tunnel: w352 -> [w356 w359 w361 w367 w368]
          tunnel: w351 -> [_ _ _ w365 _]
          tunnel: [w357 PLS_UI_State."Waiting for Exit (Acq Stopped)" ("UI State") PLS_UI_State."Waiting for Stop (Acq Stopped)" ("UI State") PLS_UI_State."Idle" ("UI State") PLS_UI_State."Idle" ("UI State")] -> w350
          tunnel: [w356 w359 w361 w366 w368] -> w349
          frame Default {
          }
          frame "Waiting for Exit", "Waiting for Exit (Acq Stopped)" {
          }
          frame "Waiting for Stop", "Waiting for Stop (Acq Stopped)" {
          }
          frame "Waiting for Exit (Log Stopped)" {
            # "If we are waiting to exit, and the logging has already stopped, then the \"Acquisition Stopped\" message indicates that it is time to exit."
            n168 = call-poly "Enqueue Message.vi"("Priority Message? (F)"=TRUE, "error in (no error)"=w367, "Message"="Exit", "Message Queue"=w365) -> ("error out"=w366:errorcluster)  [unwired: 6 in, 1 out]
          }
          frame "Waiting for Stop (Log Stopped)" {
            # "If we are waiting to stop, and the logging has already stopped, then the \"Acquisition Stopped\" message indicates that it is time to stop."
          }
        }
      }
      frame "Logging Stopped" {
        # "Logic for determining what action to take when the logging has stopped."
        n169 = case shown="\"Waiting for Exit (Acq Stopped)\"" w374 {
          selector: w374 -> [w378 _ _ _ _]
          tunnel: w373 -> [w377 w380 w382 w388 w389]
          tunnel: w372 -> [_ _ _ w386 _]
          tunnel: [w378 PLS_UI_State."Waiting for Exit (Log Stopped)" ("UI State") PLS_UI_State."Waiting for Stop (Log Stopped)" ("UI State") PLS_UI_State."Idle" ("UI State") PLS_UI_State."Idle" ("UI State")] -> w371
          tunnel: [w377 w380 w382 w387 w389] -> w370
          frame Default {
          }
          frame "Waiting for Exit", "Waiting for Exit (Log Stopped)" {
          }
          frame "Waiting for Stop", "Waiting for Stop (Log Stopped)" {
          }
          frame "Waiting for Exit (Acq Stopped)" {
            # "If we are waiting to exit, and the acquisition has already stopped, then the \"Logging Stopped\" message indicates that it is time to exit."
            n170 = call-poly "Enqueue Message.vi"("Priority Message? (F)"=TRUE, "error in (no error)"=w388, "Message"="Exit", "Message Queue"=w386) -> ("error out"=w387:errorcluster)  [unwired: 6 in, 1 out]
          }
          frame "Waiting for Stop (Acq Stopped)" {
            # "If we are waiting to stop, and the acquisition has already stopped, then the \"Logging Stopped\" message indicates that it is time to stop."
          }
        }
      }
      frame "Broadcast settings" {
        w396 = "Update Settings" ("Message")
        # "Broadcast settings - Send the 'Update Settings' message to the Logging and Acquisition message loops."
        n171 = Unbundle By Name(w408) -> ("Logging Configuration"=w398:T8, "Digital Control Configuration"=w391:T10, "Generation Settings"=w403:T9, "Acquisition Settings"=w407:T6)
        n172 = Unbundle By Name(w398) -> ("Log File Base Path"=w399:path)
        n173 = Unbundle By Name(w402) -> ("file"=w401:T26)
        n174 = Cluster To Array(cluster=w401) -> (array=w400:refnum<vi>[])
        n175 = for {
          tunnel: w400 -> [w410] mode=indexing
          tunnel: w399 -> [w409]
          n176 = property class="Path"(reference=w410, "StartPath"=w409) -> ()  [unwired: 1 in, 2 out]
        }
        n177 = call-poly "Enqueue Message.vi"("Message Data"=w407, "Message"=w396, "Message Queue"=w405) -> ("error out"=w395:errorcluster)  [unwired: 7 in, 1 out]
        n178 = call-poly "Enqueue Message.vi"("Message Data"=w403, "Message"=w396, "Message Queue"=w404) -> ("error out"=w394:errorcluster)  [unwired: 7 in, 1 out]
        n179 = call-poly "Enqueue Message.vi"("Message Data"=w391, "Message"=w396, "Message Queue"=w397) -> ("error out"=w393:errorcluster)  [unwired: 7 in, 1 out]
        n180 = Merge Errors(w393, w394, w395) -> (w392:errorcluster)
      }
      frame "Launch Settings Dialog" {
        # "Launch Settings Dialog - Launch the Settings Dialog when the user clicks the 'Settings' button."
        n181 = call "Settings Dialog.vi"("error in (no error)"=w418, "Settings in"=w419) -> ("error out"=w414:errorcluster, "Cancelled?"=w417:bool, "Settings out"=w415:T5)  [unwired: 6 in, 1 out]
        n182 = case shown="False" w417 {
          tunnel: w416 -> [w423 _]
          tunnel: w414 -> [w422 w424]
          tunnel: [w421 w424] -> w411
          frame False {
            n183 = call-poly "Enqueue Message.vi"("error in (no error)"=w422, "Message"="Broadcast Settings", "Message Queue"=w423) -> ("error out"=w421:errorcluster)  [unwired: 7 in, 1 out]
          }
          frame True {
          }
        }
      }
      frame "Error" {
        # "Always cast error data, even on incoming error."
        # "Error - Check the error message data and respond accordingly. This message is sent by the \"Error Handler\" VIs at the end of each loop in this application."
        n184 = Variant To Data(type=errorcluster {"status"=FALSE, "code"=0, "source"=""} ("error constant"), Variant=w432) -> (data=w427:errorcluster, error out=w433:errorcluster)  [unwired: 1 in]
        n185 = call <vilib>:"Simple Error Handler.vi"("error in (no error)"=w427) -> ()  [unwired: 4 in, 5 out]
        n186 = call-poly "Enqueue Message.vi"("Priority Message? (F)"=TRUE, "Message"="Exit", "Message Queue"=w431) -> ("error out"=w429:errorcluster)  [unwired: 7 in, 1 out]
        n187 = Merge Errors(w429, w433) -> (w430:errorcluster)
      }
      frame "Confirm Quit" {
        # "Confirm Quit - Message that can confirm whether or not the user wants to exit the application."
        n188 = case shown="\"Acquiring and Logging\"" w441 {
          tunnel: w440 -> [w449 w454]
          tunnel: w439 -> [w448 w453]
          tunnel: [w447 w452] -> w438
          tunnel: [PLS_UI_State."Idle" ("UI State") PLS_UI_State."Waiting for Exit" ("UI State")] -> w437
          frame Default {
            # "If 'Confirm Quit' comes in while the system is idle, there is no need for a confirmation message."
            n189 = call-poly "Enqueue Message.vi"("Priority Message? (F)"=TRUE, "error in (no error)"=w448, "Message"="Exit", "Message Queue"=w449) -> ("error out"=w447:errorcluster)  [unwired: 6 in, 1 out]
          }
          frame "Acquiring and Logging" {
            n190 = call-poly "Enqueue Message.vi"("error in (no error)"=w453, "Message"="Stop", "Message Queue"=w454) -> ("error out"=w452:errorcluster)  [unwired: 7 in, 1 out]
          }
        }
      }
      frame "Exit" {
        w455 = TRUE ("Priority Message? (F)")
        # "Stop the VI"
        # "Exit - Send Exit messages to the Acquisition and Logging loops, and fire the user event to stop the Event Handling Loop."
        n191 = call-poly "Enqueue Message.vi"("Priority Message? (F)"=w455, "Message"=w456, "Message Queue"=w460) -> ("error out"=w461:errorcluster)  [unwired: 7 in, 1 out]
        n192 = call-poly "Enqueue Message.vi"("Priority Message? (F)"=w455, "Message"=w456, "Message Queue"=w458) -> ("error out"=w462:errorcluster)  [unwired: 7 in, 1 out]
        n193 = call-poly "Enqueue Message.vi"("Priority Message? (F)"=w455, "Message"=w456, "Message Queue"=w459) -> ("error out"=w463:errorcluster)  [unwired: 7 in, 1 out]
        n194 = call-poly "Enqueue Message.vi"("Priority Message? (F)"=w455, "Message"=w456, "Message Queue"=w457) -> ("error out"=w464:errorcluster)  [unwired: 7 in, 1 out]
        n195 = Merge Errors(w464, w463, w462, w461) -> (w465:errorcluster)
        n196 = call "Fire User Event - Stop.vi"("error in (no error)"=w465, "User Event - Stop"=w470) -> ("error out"=w469:errorcluster)  [unwired: 9 in]
      }
      frame "---Copy This Frame---" {
        # "Duplicate this frame when creating new messages.  Change this comment in the duplicated frame to describe this message."
        n197 = Merge Errors(w476) -> (w475:errorcluster)
      }
      frame "port" {
        # "control vannes"
        n198 = call-poly "Enqueue Message.vi"("error in (no error)"=w478, "Message Data"=w479, "Message"=w480, "Message Queue"=w477) -> ("error out"=w482:errorcluster)  [unwired: 6 in, 1 out]
      }
      frame "setpoint" {
        # "nouvelle consigne de température"
        n199 = call-poly "Enqueue Message.vi"("error in (no error)"=w486, "Message Data"=w487, "Message"=w488, "Message Queue"=w485) -> ("error out"=w490:errorcluster)  [unwired: 6 in, 1 out]
      }
      frame Default {
        # "'Default' case only runs if there is a message that isn't defined in any of the other cases.  Output a programming error."
        n200 = xnode "Error Ring"("parameter 0"=w494) -> ("error out"=w493:errorcluster)
      }
    }
    n201 = call "PLS Error Handler - Message Handling Loop.vi"("error in (no error)"=w162, "Message Queue"=w161) -> ("dup error in"=w163:errorcluster)  [unwired: 8 in, 1 out]
  }
  n202 = call "Acquisition Message Loop.vi"("error in (no error)"=w3, "Data Queue"=w11, "Data Notifier"=w12, "Message Queues"=w4) -> ("error out"=w27:errorcluster)  [unwired: 7 in]
  n203 = call "Logging Message Loop.vi"("error in (no error)"=w3, "Data Queue"=w11, "Message Queues"=w4) -> ("error out"=w9:errorcluster)  [unwired: 8 in]
  n204 = call "Generation Message Loop.vi"("error in (no error)"=w3, "Data Notifier"=w12, "Message Queues"=w4) -> ("error out"=w8:errorcluster)  [unwired: 8 in]
  n205 = call "Digital Control Loop.vi"("error in (no error)"=w3, "Message Queues"=w4) -> ("error out"=w2:errorcluster)  [unwired: 9 in]
  n206 = Unregister For Events(event registration refnum=w23, error in=w28) -> (error out=w24:errorcluster)
  n207 = Release Queue(queue=w18, error in (no error)=w29) -> (error out=w16:errorcluster)  [unwired: 1 in, 2 out]
  n208 = Release Queue(queue=w11, error in (no error)=w16) -> (error out=w15:errorcluster)  [unwired: 1 in, 2 out]
  n209 = Release Notifier(notifier=w12, error in (no error)=w15) -> (error out=w14:errorcluster)  [unwired: 1 in, 2 out]
  n210 = Merge Errors(w24, w14, w27, w9, w8, w2) -> (w19:errorcluster)
  n211 = call "Destroy User Event - Stop.vi"("error in (no error)"=w19, "User Event - Stop"=w1) -> ("error out"=w17:errorcluster)  [unwired: 9 in]
  n212 = disable-structure shown="RUN_TIME_ENGINE==True" {
    disable-tunnel: w17 -> [_ _]
    frame condition #0 (active) {
    }
    frame condition #1 {
      # "Call Quit LabVIEW if running as a built application."
      n213 = Quit LabVIEW() -> ()  [unwired: 1 in]
    }
  }
